vi "Butterfly Graph.vi"() -> ()   [LabVIEW 2012]
uses:
  <vilib>/gmath/NI_Gmath.lvlib
panel:
  in  "radius as function of angle":string="exp(cos(t))-2*cos(4*t)+sin(t/12)^5" caption="极径（极角的函数）"
  out "error":i32 caption="错误"
  in  "number of points":u32=2000 caption="点数"
  in  "end":dbl=45.0 caption="结束" format="%.2f"
  in  "start":dbl caption="开始" format="%.2f"
  out "Lissajous  Graph":T1(graph)
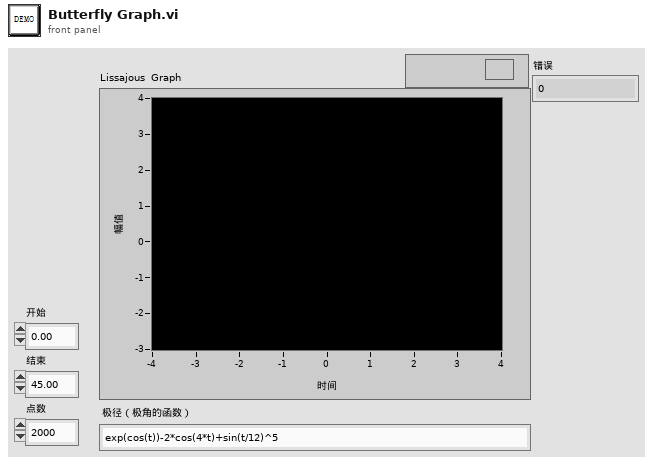
[diagram p1: front panel]
types:
  T1 = cluster{"Sinusoidal Pattern":dbl[], "Sinusoidal Pattern":dbl[]}
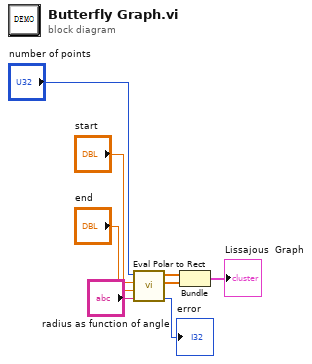
[diagram p0: block diagram]
diagram:
  n1 = call <vilib>:"Eval Polar to Rect.vi"("radius as function of angle"="radius as function of angle", "end"="end", "start"="start", "number of points"="number of points") -> ("error"=→"error":i32, "Y"=w2:dbl[], "X"=w6:dbl[])  [unwired: 1 out]
  n2 = Bundle("X"=w6, "Y"=w2) -> (→"Lissajous  Graph":cluster{"X":dbl[], "Y":dbl[]})  [unwired: 1 in]
